vi "CHANNEL.vi"() -> ()   [LabVIEW 2013]
uses:
  Global.vi
panel:
  out "Channel Log":variant=variant("A"=variant(dbl 4.0), "B"=variant(dbl 5.0), "C"=variant(dbl 6.0))
  in  "Channel":string="C"
  out "Options":string="C"
  in  "stop":bool
  out "VAR index":i32
  out "Val":dbl=6.0 format="%.2f"
  out "Set":bool
  out "Recieved":bool
  in  "Var":string="CHAN"
  # "Sets the output of a multi-\nchannel voltage supply.\n\nValue Type: DBL\nOptions: channel name"
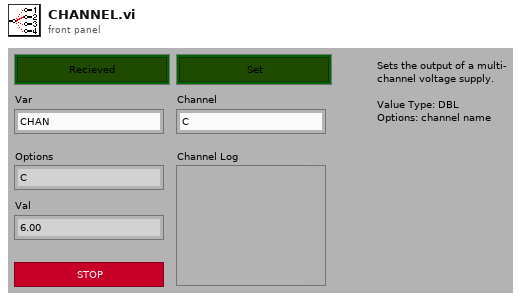
[diagram p1: front panel]
types:
  T1 = typedef "Semaphore RefNum" = refnum<k1>
  T2 = cluster{"VAR":string, "Options":string, "Val":string, "Recieved":bool, "Set":bool}[]
  T3 = cluster{"VAR":string, "Options":string, "Val":string, "Recieved":bool, "Set":bool}
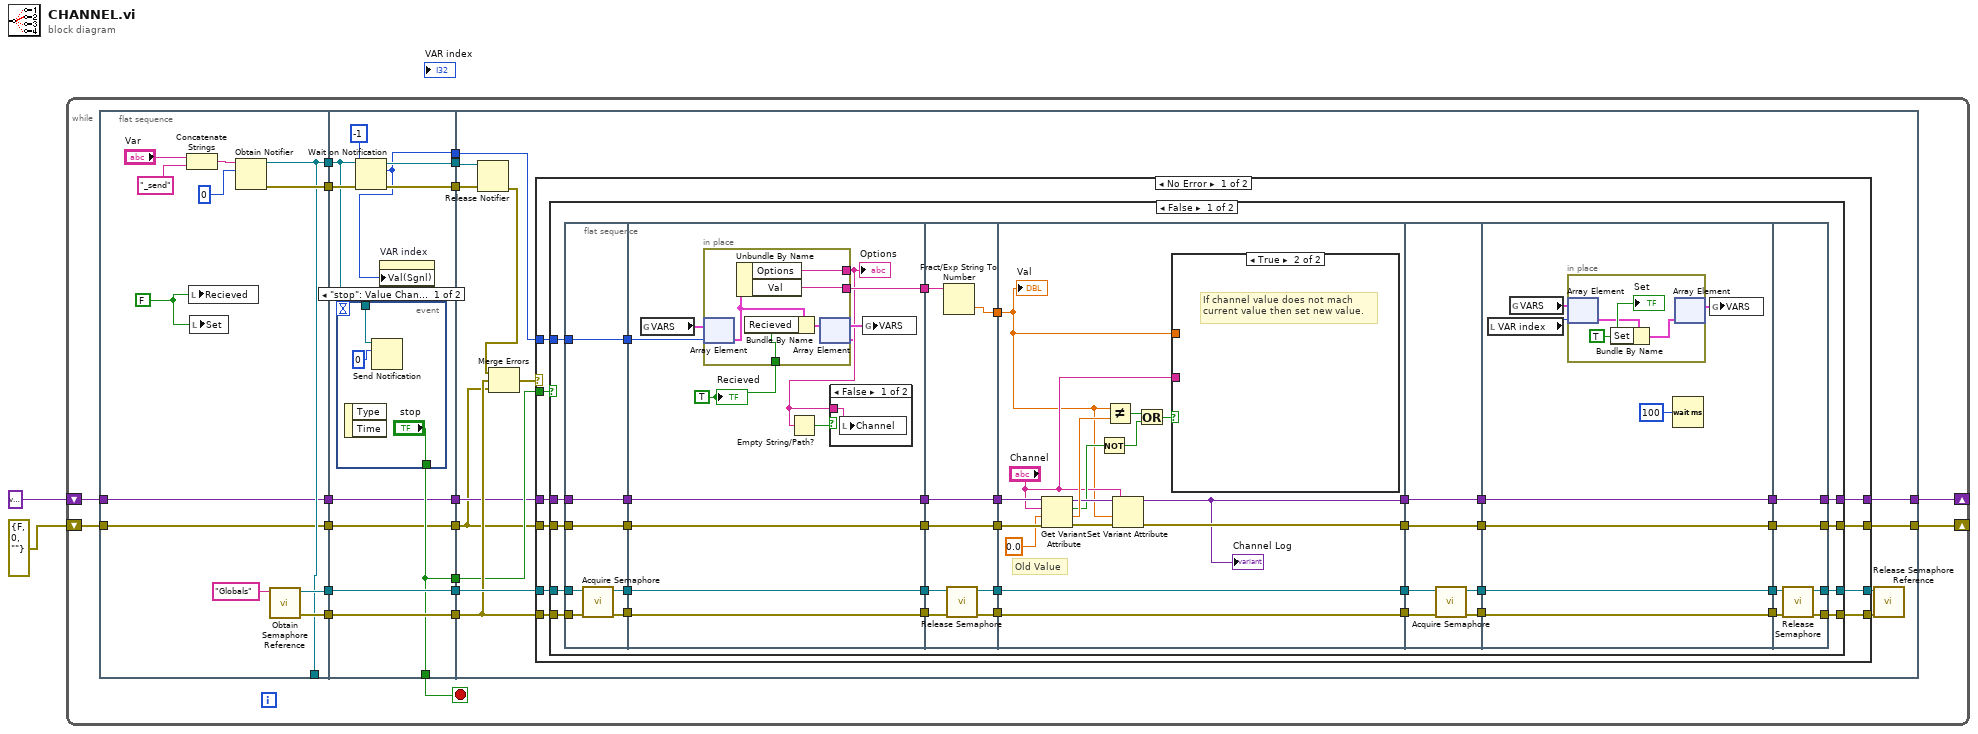
[diagram p0: block diagram]
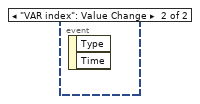
[diagram p2: hidden frame]
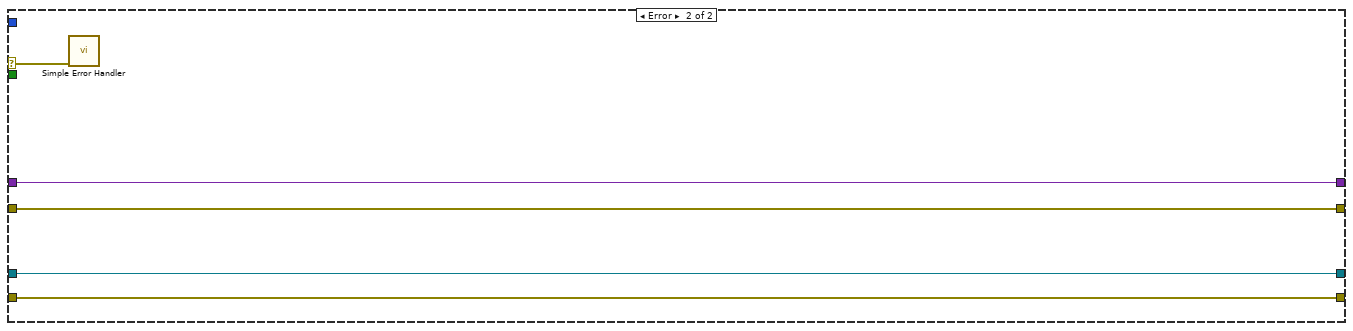
[diagram p6: hidden frame]
diagram:
  n1 = while {
    shift-right: [w3] -> _
    shift-left: variant -> [w8]
    shift-right: [w4] -> _
    shift-left: errorcluster {"status"=FALSE, "code"=0, "source"=""} ("error out") -> [w5]
    stop <- w12 stop-if-true
    n2 = flat-sequence {
      tunnel: [w25] -> w21
      tunnel: [w24] -> w20
      tunnel: [w31] -> w16
      tunnel: [w30] -> w14
      tunnel: [w24] -> _
      tunnel: [w23] -> w9
      tunnel: w8 -> [w23]
      tunnel: [w22] -> w6
      tunnel: w5 -> [w22]
      tunnel: w21 -> [w43]
      tunnel: w20 -> [w37]
      tunnel: [w42] -> w19
      tunnel: [w39] -> w18
      tunnel: [w38] -> w17
      tunnel: w16 -> [w41]
      tunnel: [w41] -> w15
      tunnel: w14 -> [w40]
      tunnel: [w40] -> w13
      tunnel: [w36] -> w12
      tunnel: [w36] -> w11
      tunnel: [w35] -> w10
      tunnel: w9 -> [w35]
      tunnel: [w34] -> w7
      tunnel: w6 -> [w34]
      tunnel: w19 -> [w54]
      tunnel: w18 -> [w55]
      tunnel: w17 -> [w61]
      tunnel: w15 -> [w60]
      tunnel: w13 -> [w57]
      tunnel: w11 -> [w52]
      tunnel: w10 -> [w51]
      tunnel: w7 -> [w50]
      tunnel: [w49] -> w4
      tunnel: [w48] -> w3
      frame #0 {
        w33 = FALSE ("notification")
        n3 = Concatenate Strings("Var", "_send") -> (w28:string)
        n4 = local write "Recieved"(w33) -> ()
        n5 = local write "Set"(w33) -> ()
        n6 = Obtain Notifier(name (unnamed)=w28, notification data type=0) -> (notifier out=w24:refnum<notifier>, error out=w25:errorcluster)  [unwired: 2 in, 1 out]
        n7 = call <vilib>:"Obtain Semaphore Reference.vi"("name (unnamed)"="Globals") -> ("error out"=w30:errorcluster, "semaphore"=w31:T1)  [unwired: 4 in, 1 out]
      }
      frame #1 {
        n8 = event shown="[0] \"stop\": Value Change" {
          selector: _ -> [_ _]
          dyn-events: _ -> [_ _]
          timeout: _ -> [_ _]
          tunnel: ["stop" _] -> w36
          tunnel: w37 -> [w46 _]
          event "stop": Value Change {
            n9 = event-data() -> ()  [unwired: 1 in, 2 out]
            n10 = Send Notification(notification=0, notifier=w46) -> ()  [unwired: 1 in, 2 out]
          }
          event "VAR index": Value Change {
            n11 = event-data() -> ()  [unwired: 1 in, 2 out]
          }
        }
        n12 = Wait on Notification(notifier=w37, timeout in ms (-1)=-1, error in (no error)=w43) -> (notifier out=w42:refnum<notifier>, notification=w38:i32, error out=w39:errorcluster)  [unwired: 1 in, 1 out]
        n13 = property on="VAR index" class="DigNum (strict)"("Val(Sgnl)"=w38) -> ()  [unwired: 2 in, 2 out]
      }
      frame #2 {
        n14 = Release Notifier(notifier=w54, error in (no error)=w55) -> (error out=w53:errorcluster)  [unwired: 1 in, 2 out]
        n15 = Merge Errors(w53, w57, w50) -> (w56:errorcluster)
        n16 = case shown="No Error" w56 {
          selector: w56 -> [_ w185]
          tunnel: w61 -> [w71 _]
          tunnel: w60 -> [w70 w187]
          tunnel: w57 -> [w69 w186]
          tunnel: [w68 w186] -> w59
          tunnel: [w67 w187] -> w58
          tunnel: w52 -> [w66 _]
          tunnel: w51 -> [w65 w184]
          tunnel: w50 -> [w64 w183]
          tunnel: [w63 w183] -> w49
          tunnel: [w62 w184] -> w48
          frame No Error {
            n17 = case shown="False" w66 {
              tunnel: w71 -> [w93 _]
              tunnel: w70 -> [w92 w182]
              tunnel: w69 -> [w91 w181]
              tunnel: [w90 w181] -> w68
              tunnel: [w89 w182] -> w67
              tunnel: w65 -> [w86 w180]
              tunnel: w64 -> [w83 w179]
              tunnel: [w78 w179] -> w63
              tunnel: [w73 w180] -> w62
              frame False {
                n18 = flat-sequence {
                  tunnel: w91 -> [w112]
                  tunnel: w92 -> [w113]
                  tunnel: w93 -> [w114]
                  tunnel: [w114] -> w107
                  tunnel: [w111] -> w106
                  tunnel: [w110] -> w105
                  tunnel: [w109] -> w87
                  tunnel: w86 -> [w109]
                  tunnel: [w108] -> w84
                  tunnel: w83 -> [w108]
                  tunnel: w107 -> [w120]
                  tunnel: w106 -> [w124]
                  tunnel: w105 -> [w125]
                  tunnel: [w125] -> w104
                  tunnel: [w124] -> w103
                  tunnel: [w119] -> w102
                  tunnel: [w118] -> w88
                  tunnel: w87 -> [w118]
                  tunnel: [w117] -> w85
                  tunnel: w84 -> [w117]
                  tunnel: w104 -> [w138]
                  tunnel: w103 -> [w139]
                  tunnel: [w137] -> w101
                  tunnel: [w136] -> w100
                  tunnel: w102 -> [w133]
                  tunnel: w88 -> [w134]
                  tunnel: w85 -> [w135]
                  tunnel: [w135] -> w79
                  tunnel: [w134] -> w75
                  tunnel: [w132] -> w72
                  tunnel: w101 -> [w155]
                  tunnel: w100 -> [w154]
                  tunnel: [w155] -> w99
                  tunnel: [w154] -> w98
                  tunnel: [w147] -> w80
                  tunnel: w79 -> [w152]
                  tunnel: [w146] -> w76
                  tunnel: w75 -> [w153]
                  tunnel: w72 -> [w140]
                  tunnel: w99 -> [w161]
                  tunnel: w98 -> [w158]
                  tunnel: [w160] -> w97
                  tunnel: [w159] -> w96
                  tunnel: [w157] -> w81
                  tunnel: w80 -> [w157]
                  tunnel: [w156] -> w77
                  tunnel: w76 -> [w156]
                  tunnel: [w169] -> w95
                  tunnel: w97 -> [w169]
                  tunnel: [w165] -> w94
                  tunnel: w96 -> [w165]
                  tunnel: [w164] -> w82
                  tunnel: w81 -> [w164]
                  tunnel: w77 -> [w163]
                  tunnel: [w163] -> w74
                  tunnel: w95 -> [w178]
                  tunnel: w94 -> [w177]
                  tunnel: [w176] -> w90
                  tunnel: [w175] -> w89
                  tunnel: w82 -> [w174]
                  tunnel: [w174] -> w78
                  tunnel: w74 -> [w173]
                  tunnel: [w173] -> w73
                  frame #0 {
                    n19 = call <vilib>:"Acquire Semaphore.vi"("error in (no error)"=w112, "semaphore"=w113) -> ("error out"=w111:errorcluster, "semaphore out"=w110:T1)  [unwired: 3 in, 1 out]
                  }
                  frame #1 {
                    w121 = TRUE ("Found")
                    n20 = global read "Global.vi" "VARS"() -> (w122:T2)
                    n21 = in-place {
                      in-place-border: [w129] -> w119
                      in-place-border: w121 -> [w128]
                      in-place-border: [w127] -> w116
                      n22 = in-place-array #1(w122, w120) -> (w131:T3)
                      n23 = Unbundle By Name(w131) -> ("Options"=w127:string, "Val"=w129:string)
                      n24 = Bundle By Name(cluster=w131, "Recieved"=w128) -> (w130:T3)
                      n25 = in-place-array #1(w130) -> (w123:T2)  [unwired: 1 out]
                    }
                    "Options" <- w116
                    n26 = Empty String/Path?(string/path=w116) -> (empty?=w115:bool)
                    n27 = case shown="False" w115 {
                      tunnel: w116 -> [w126 _]
                      frame False {
                        n28 = local write "Channel"(w126) -> ()
                      }
                      frame True {
                      }
                    }
                    n29 = global write "Global.vi" "VARS"(w123) -> ()
                    "Recieved" <- w121
                  }
                  frame #2 {
                    n30 = Fract/Exp String To Number(string=w133) -> (number=w132:dbl)  [unwired: 3 in, 1 out]
                    n31 = call <vilib>:"Release Semaphore.vi"("error in (no error)"=w139, "semaphore"=w138) -> ("error out"=w136:errorcluster, "semaphore out"=w137:T1)  [unwired: 4 in]
                  }
                  frame #3 {
                    # "Old Value"
                    n32 = Get Variant Attribute(Variant=w153, name="Channel", default value (empty Variant)=0.0, error in=w152) -> (duplicate Variant=w149:variant, found=w143:bool, value=w150:dbl, error out=w148:errorcluster)
                    n33 = Not(x=w143) -> (.not. x?=w144:bool)
                    n34 = Not Equal?(x=w140, y=w150) -> (x != y?=w145:bool)
                    n35 = Set Variant Attribute(Variant=w149, name="Channel", value=w140, error in=w148) -> (Variant out=w146:variant, error out=w147:errorcluster)  [unwired: 1 out]
                    "Channel Log" <- w146
                    n36 = Or(x=w145, y=w144) -> (x .or. y?=w142:bool)
                    n37 = case shown="True" w142 {
                      tunnel: w140 -> [_ _]
                      tunnel: "Channel" -> [_ _]
                      frame False {
                      }
                      frame True {
                        # "If channel value does not mach \ncurrent value then set new value."
                      }
                    }
                    "Val" <- w140
                  }
                  frame #4 {
                    n38 = call <vilib>:"Acquire Semaphore.vi"("error in (no error)"=w158, "semaphore"=w161) -> ("error out"=w159:errorcluster, "semaphore out"=w160:T1)  [unwired: 3 in, 1 out]
                  }
                  frame #5 {
                    n39 = local read "VAR index"() -> (w168:i32)
                    n40 = global read "Global.vi" "VARS"() -> (w167:T2)
                    n41 = in-place {
                      w172 = TRUE ("Set")
                      n42 = in-place-array #2(w167, w168) -> (w171:T3)
                      n43 = Bundle By Name(cluster=w171, "Set"=w172) -> (w170:T3)
                      n44 = in-place-array #2(w170) -> (w166:T2)  [unwired: 1 out]
                      "Set" <- w172
                    }
                    n45 = Wait (ms)(milliseconds to wait=u32 100) -> ()  [unwired: 1 out]
                    n46 = global write "Global.vi" "VARS"(w166) -> ()
                  }
                  frame #6 {
                    n47 = call <vilib>:"Release Semaphore.vi"("error in (no error)"=w177, "semaphore"=w178) -> ("error out"=w176:errorcluster, "semaphore out"=w175:T1)  [unwired: 4 in]
                  }
                }
              }
              frame True {
              }
            }
          }
          frame Error {
            n48 = call <vilib>:"Simple Error Handler.vi"("error in (no error)"=w185) -> ()  [unwired: 4 in, 5 out]
          }
        }
        n49 = call <vilib>:"Release Semaphore Reference.vi"("error in (no error)"=w59, "semaphore"=w58) -> ()  [unwired: 8 in, 2 out]
      }
    }
  }
